vi "TCP-IP.ping.vi"(8 "error in (no error)":errorcluster caption="错误输入（无错误）", 11 "IP Address":string) -> (0 "error out":errorcluster caption="错误输出", 2 "standard output":string caption="标准输出", 3 "ok?":bool)   [LabVIEW 2012, in "Lib_UEL.ATE.lvlib" / "Lib_IPVoice.lvlib"]
uses:
  <vilib>/regexp/Match Regular Expression.xnode
  Lib_IPVoice.lvlib
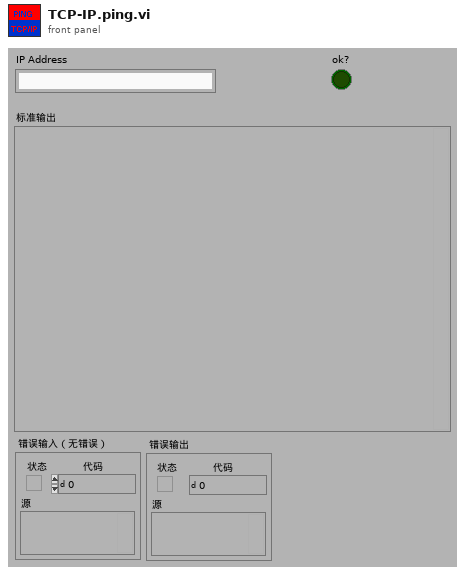
[diagram p1: front panel]
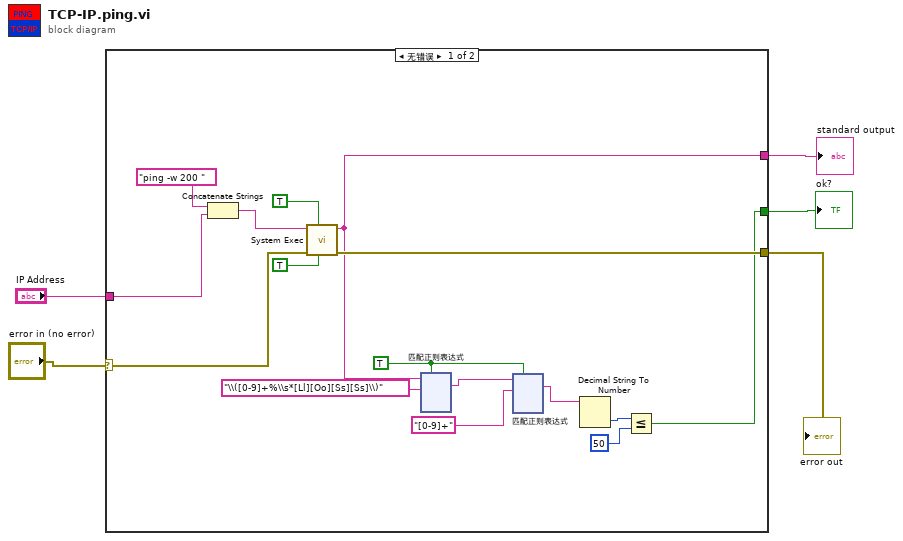
[diagram p0: block diagram]
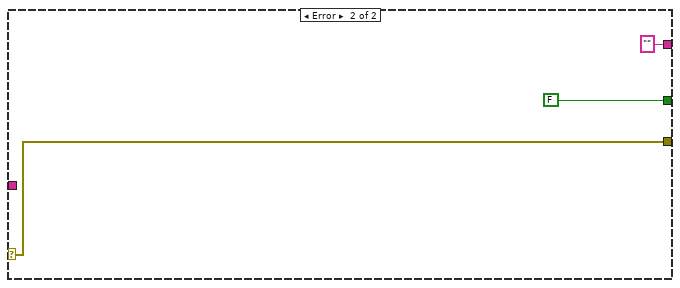
[diagram p2: hidden frame]
diagram:
  n1 = case shown="无错误" "error in (no error)" {
    selector: "error in (no error)" -> [w15 w246]
    tunnel: "IP Address" -> [w18 _]
    tunnel: [w16 w246] -> w4
    tunnel: [w7 FALSE ("ok?")] -> w2
    tunnel: [w14 "" ("standard output")] -> w1
    frame No Error {
      w12 = TRUE ("忽略大小写？(F)")
      n2 = Concatenate Strings("ping -w 200 " ("command line"), w18) -> (w17:string)
      n3 = call <vilib>:"System Exec.vi"("run minimized? (F)"=TRUE, "wait until completion? (T)"=TRUE, "error in (no error)"=w15, "command line"=w17) -> ("error out"=w16:errorcluster, "standard output"=w14:string)  [unwired: 4 in, 2 out]
      n4 = xnode "匹配正则表达式"("输入字符串"=w14, "正则表达式"="\\([0-9]+%\\s*[Ll][Oo][Ss][Ss]\\)", "忽略大小写？(F)"=w12) -> ("所有匹配"=w11:string)  [unwired: 3 in, 4 out]
      n5 = xnode "匹配正则表达式"("输入字符串"=w11, "正则表达式"="[0-9]+", "忽略大小写？(F)"=w12) -> ("所有匹配"=w9:string)  [unwired: 3 in, 4 out]
      n6 = Decimal String To Number(string=w9) -> (number=w6:i32)  [unwired: 2 in, 1 out]
      n7 = Less Or Equal?(x=w6, y=50) -> (x <= y?=w7:bool)
    }
    frame Error {
    }
  }
  "error out" <- w4
  "ok?" <- w2
  "standard output" <- w1
